vi "Script Logging.vi"(8 "error in (no error)":errorcluster, 11 "custom device":T1 format="%.0x") -> (0 "error out":errorcluster, 2 "RT log file path":string, 3 "custom device out":T1 format="%.0x")   [LabVIEW 2020]
uses:
  <vilib>/NI VeriStand/Custom Device API/Custom Device Item Ref.ctl
  Scripting/AIM MIL-STD-1553 Scripting.lvlib
  <vilib>/NI VeriStand/Custom Device API/Custom Device API.lvlib
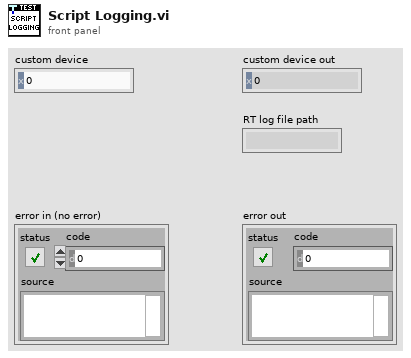
[diagram p1: front panel]
types:
  T1 = typedef "Custom Device API.lvlib/Custom Device Item Ref.ctl" = u64
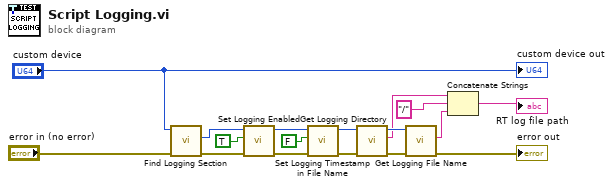
[diagram p0: block diagram]
diagram:
  n1 = call "Find Logging Section.vi"("error in"="error in (no error)", "custom device"="custom device") -> ("error out"=w9:errorcluster, "logging section"=w13:T1)  [unwired: 7 in, 1 out]
  n2 = call "Set Logging Enabled.vi"("error in"=w9, "logging enabled"=TRUE, "logging section"=w13) -> ("error out"=w8:errorcluster, "logging section out"=w11:T1)  [unwired: 7 in]
  n3 = call "Set Logging Timestamp in File Name.vi"("error in"=w8, "timestamp in file name"=FALSE, "logging section"=w11) -> ("error out"=w6:errorcluster, "logging section out"=w7:T1)  [unwired: 7 in]
  n4 = call "Get Logging Directory.vi"("error in"=w6, "logging section"=w7) -> ("error out"=w15:errorcluster, "directory"=w3:string, "logging section out"=w14:T1)  [unwired: 7 in]
  n5 = call "Get Logging File Name.vi"("error in"=w15, "logging section"=w14) -> ("error out"=→"error out":errorcluster, "file name"=w2:string)  [unwired: 7 in, 1 out]
  n6 = Concatenate Strings(w3, "/" ("string"), w2) -> (→"RT log file path":string)
  "custom device out" <- "custom device"
